vi "Add(TimeStamp+ms).vi"(1 "Enable(T)":bool=TRUE, 2 "In":timestamp, 4 "n":dbl[unit]=0.001) -> (6 "Out":timestamp)   [LabVIEW 2013]
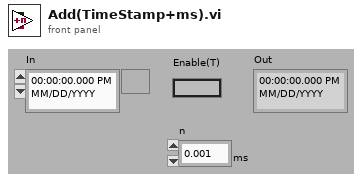
[diagram p1: front panel]
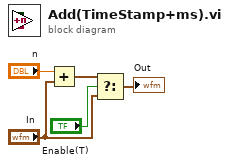
[diagram p0: block diagram]
diagram:
  n1 = Add(x="n", y="In") -> (x+y=w1:timestamp)
  n2 = Select(t=w1, s="Enable(T)", f="In") -> (s? t:f=→"Out":timestamp)
